vi "Write Channel Ring.vi"(8 "error in":errorcluster, 10 "Channel Ring":refnum<vi>, 11 "PowerSupply in":refnum<class "PowerSupply.lvclass">) -> (0 "error out":errorcluster, 3 "PowerSupply out":refnum<class "PowerSupply.lvclass">)   [LabVIEW 2019, in "PowerSupply.lvlib" / "PowerSupply.lvclass"]
uses:
  Library/PowerSupply.lvclass
  Library/PowerSupply.lvclass/PowerSupply.ctl
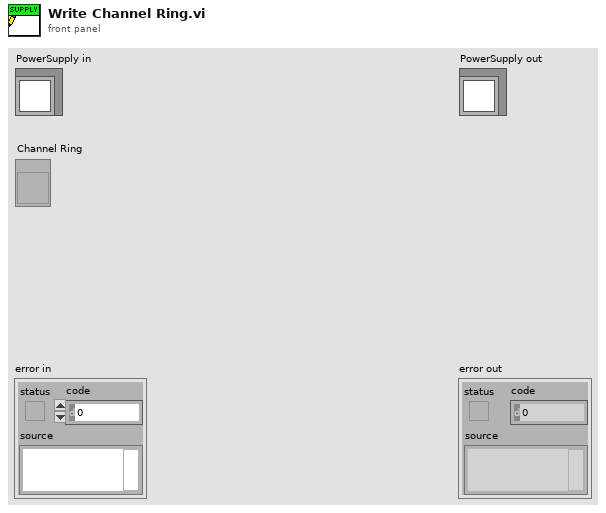
[diagram p1: front panel]
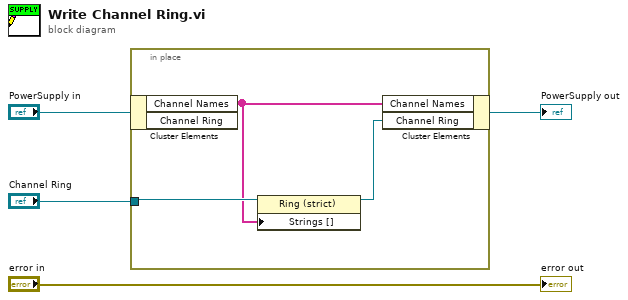
[diagram p0: block diagram]
diagram:
  n1 = in-place {
    in-place-border: "Channel Ring" -> [w7]
    n2 = in-place-cluster #1("PowerSupply in") -> ("Channel Names"=w5:string[])  [unwired: 1 out]
    n3 = property class="Ring (strict)"(reference=w7, "Strings []"=w5) -> (reference out=w6:refnum<vi>)  [unwired: 1 in, 1 out]
    n4 = in-place-cluster #1("Channel Names"=w5, "Channel Ring"=w6) -> (→"PowerSupply out":refnum<class "PowerSupply.lvclass">)
  }
  "error out" <- "error in"
